vi "PicoScope4000ExampleStreaming.vi"() -> ()   [LabVIEW 2015]
panel:
  in  "Trigger Settings":T1={"Trigger Enabled"=TRUE, "Trigger Source"=enum."Channel A", "Trigger Threshold (16-bit counts)"=0, "Trigger Direction"=2, "Trigger Delay (samples)"=0, "Auto Trigger Time (ms)"=1000, "PicoScope 4262 Ext. Trigger Range"=5} {"PicoScope 4262 Ext. Trigger Range" items=["500 mV"=5, "5 V"=8]; "Trigger Direction" items=["Rising"=2, "Falling"=3]}
  out "Unit Info":T2
  out "Auto Stopped":bool
  out "Triggered":bool
  out "Total Samples":u32
  in  "Acquisition Settings":T3={"Auto Stop"=TRUE, "Four Channel Device?"=FALSE, "Desired Sample Interval"=1, "Pre-trigger Samples"=0, "Post-trigger Samples"=1000000, "Down-Sample Ratio"=1, "Temp Buffer Size"=50000, "Time Units"=3} {"Time Units" items=["Nanoseconds (ns)"=2, "Microseconds (us)"=3, "Milliseconds (ms)"=4, "Seconds (s)"=5]}
  out "Sample Interval":u32=1
  in  "Apply Settings":bool
  in  "Channel A Settings":T4={"Enabled"=TRUE, "DC Coupled"=TRUE, "Range"=6} {"Range" items=["10 mV", "20 mV", "50 mV", "100 mV", "200 mV", "500 mV", "1 V", "2 V", "5 V", "10 V", "20 V", "50 V ", "100 V"]}
  out "Channel A":i16[](graph)
  in  "stop":bool
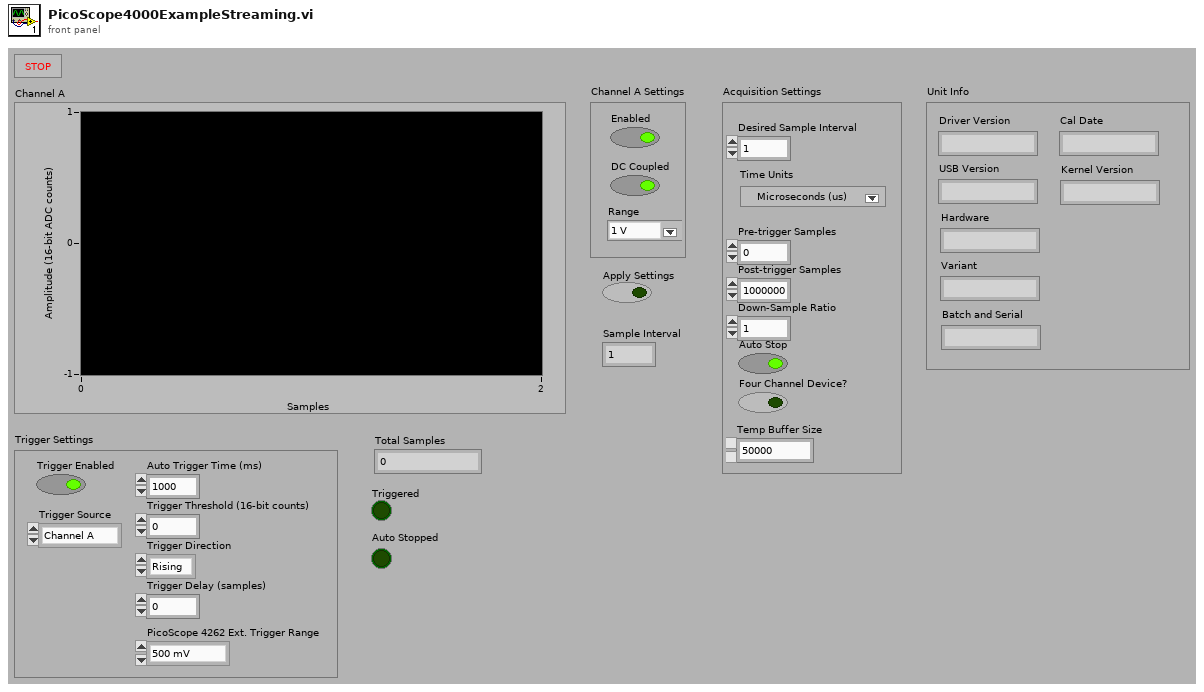
[diagram p1: front panel]
types:
  T1 = cluster{"Trigger Enabled":bool, "Trigger Source":enum32{"Channel A", "Channel B", "Channel C", "Channel D", "External"}, "Trigger Threshold (16-bit counts)":i16, "Trigger Direction":u32, "Trigger Delay (samples)":u32, "Auto Trigger Time (ms)":i16, "PicoScope 4262 Ext. Trigger Range":u32}
  T2 = cluster{"Driver Version":string, "USB Version":string, "Hardware":string, "Variant":string, "Batch and Serial":string, "Cal Date":string, "Kernel Version":string}
  T3 = cluster{"Auto Stop":bool, "Four Channel Device?":bool, "Desired Sample Interval":u32, "Pre-trigger Samples":u32, "Post-trigger Samples":u32, "Down-Sample Ratio":u32, "Temp Buffer Size":i32, "Time Units":u32}
  T4 = cluster{"Enabled":bool, "DC Coupled":bool, "Range":u16}
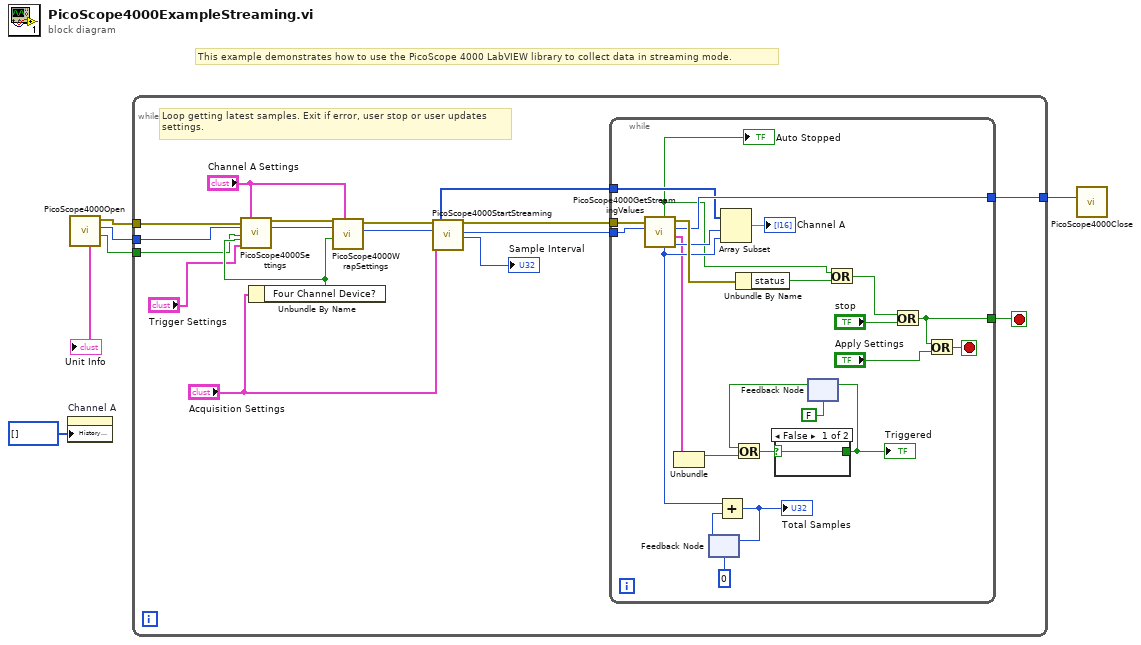
[diagram p0: block diagram]
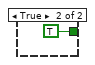
[diagram p2: hidden frame]
diagram:
  # "This example demonstrates how to use the PicoScope 4000 LabVIEW library to collect data in streaming mode."
  n1 = property on="Channel A" class="WFChart (strict)"("History Data"=i16[] []) -> ()  [unwired: 2 in, 2 out]
  n2 = call "PicoScope4000Open.vi"() -> ("Unit Info"=→"Unit Info":T2, "PicoScope 4262?"=w1:bool, "handle"=w5:i16, "error out"=w6:errorcluster)  [unwired: 4 in]
  n3 = while {
    tunnel: [w23] -> w4
    tunnel: w6 -> [w22]
    tunnel: w5 -> [w21]
    tunnel: w1 -> [w7]
    stop <- w20 stop-if-true
    # "Loop getting latest samples. Exit if error, user stop or user updates \nsettings."
    n4 = Unbundle By Name("Acquisition Settings") -> ("Four Channel Device?"=w11:bool)
    n5 = call "PicoScope4000Settings.vi"("error in"=w22, "Channel A Settings"="Channel A Settings", "handle in"=w21, "PicoScope 4262?"=w7, "Four Channel Device?"=w11, "Trigger Settings"="Trigger Settings") -> ("error out"=w13:errorcluster, "handle out"=w14:i16)  [unwired: 8 in]
    n6 = call "PicoScope4000WrapSettings.vi"("Channel A Settings"="Channel A Settings", "Four Channel Device?"=w11, "Handle In"=w14, "error in (no error)"=w13) -> ("Handle Out"=w15:i16, "error out"=w12:errorcluster)  [unwired: 6 in]
    n7 = call "PicoScope4000StartStreaming.vi"("error in"=w12, "handle in"=w15, "Acquisition Settings"="Acquisition Settings") -> ("Channel A"=w18:i16[], "error out"=w19:errorcluster, "handle out"=w17:i16, "Sample Interval"=→"Sample Interval":u32)  [unwired: 10 in, 3 out]
    n8 = while {
      tunnel: w19 -> [w44]
      tunnel: [w45] -> w23
      tunnel: [w42] -> w20
      tunnel: w18 -> [w40]
      tunnel: w17 -> [w37]
      stop <- w41 stop-if-true
      n9 = call "PicoScope4000GetStreamingValues.vi"("handle in"=w37, "error in"=w44) -> ("Start Index"=w39:u32, "Trigger"=w28:cluster{bool, "triggeredAt":u32}, "handle out"=w45:i16, "error out"=w46:errorcluster, "Number of Samples"=w33:i32, "Auto Stopped"=w24:bool)  [unwired: 4 in]
      "Auto Stopped" <- w24
      n10 = Unbundle(w28) -> (w29:bool)  [unwired: 1 out]
      n11 = feedback #1(u32 0) -> (w35:u32)
      n12 = Add(x=w33, y=w35) -> (x+y=w34:u32)
      "Total Samples" <- w34
      n13 = feedback-in #1(w34) -> ()
      n14 = Array Subset(array=w40, index=w39, length=w33) -> (→"Channel A":i16[])
      n15 = Unbundle By Name(w46) -> ("status"=w25:bool)
      n16 = feedback #2(FALSE) -> (w32:bool)
      n17 = Or(x=w32, y=w29) -> (x .or. y?=w31:bool)
      n18 = case shown="False" w31 {
        selector: w31 -> [w48 _]
        tunnel: [w48 TRUE] -> w27
        frame False {
        }
        frame True {
        }
      }
      "Triggered" <- w27
      n19 = feedback-in #2(w27) -> ()
      n20 = Or(x=w24, y=w25) -> (x .or. y?=w26:bool)
      n21 = Or(x=w26, y="stop") -> (x .or. y?=w42:bool)
      n22 = Or(x=w42, y="Apply Settings") -> (x .or. y?=w41:bool)
    }
  }
  n23 = call "PicoScope4000Close.vi"("handle"=w4) -> ()
